vi "SerialPort_MicroZed.vi"(2 "error in (no error)":errorcluster, 3 "COM Port":refnum<visa-resource-name>="COM4") -> (0 "error out":errorcluster)   [LabVIEW 2014]
uses:
  <vilib>/Instr/_visa.llb/VISA Open Access Mode.ctl
  <vilib>/Instr/_visa.llb/VISA Configure Serial Port (Instr).vi
  g_Stop.vi
  g_MicroZed_Interface.vi
  g_ReportControl.vi
panel:
  out "sent":string
  out "Terminal":string
  out "Write":string
  out "read buffer":string
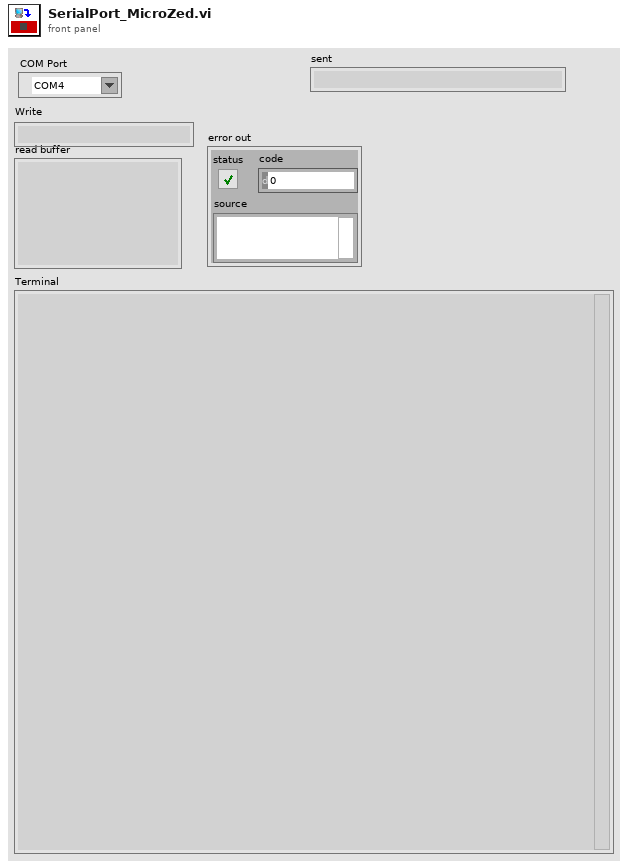
[diagram p1: front panel]
types:
  T1 = typedef "VISA Open Access Mode.ctl" = u32
  T2 = typedef "c_MicroZedInstr_Enum.ctl" = enum16{"Start Test Procedure", "Print Instructions", "Config HCC Register", "Send Parameters"}
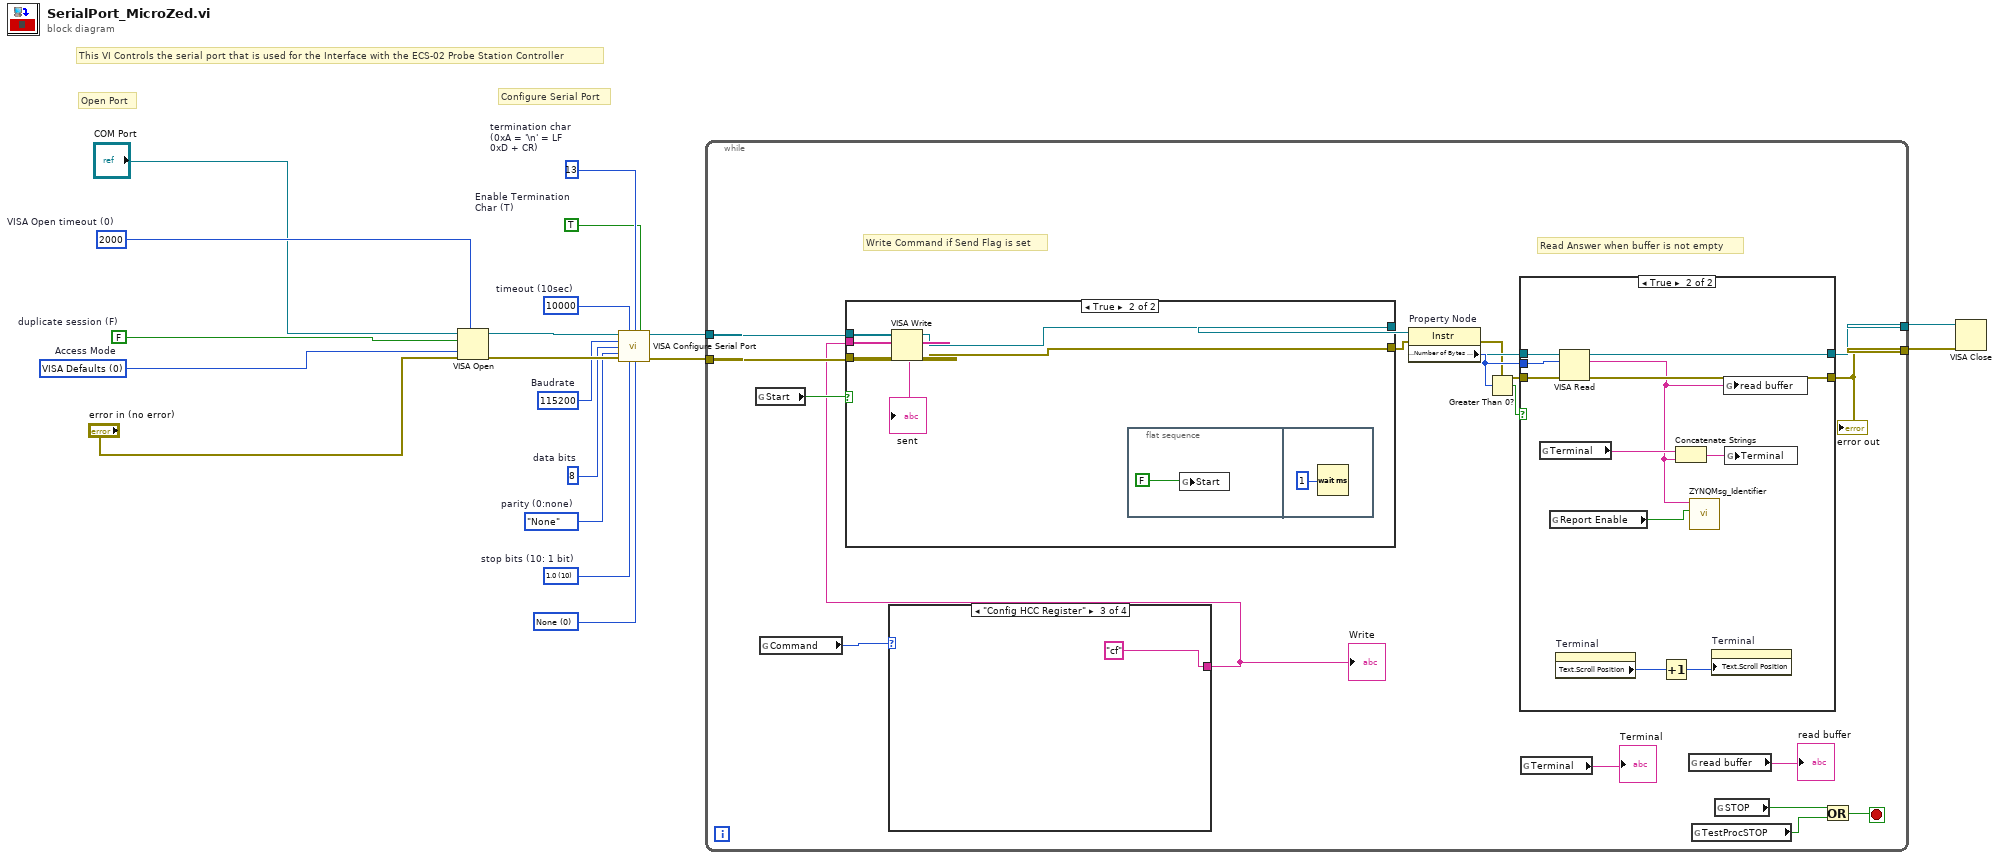
[diagram p0: block diagram]
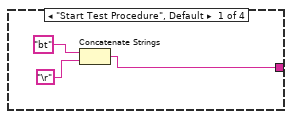
[diagram p2: hidden frame]
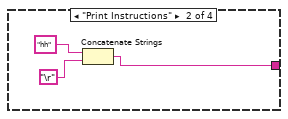
[diagram p3: hidden frame]
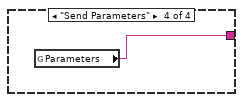
[diagram p4: hidden frame]
diagram:
  w5 = u32 10000  # timeout (10sec)
  w6 = T1 0 items=["VISA Defaults"=0, "Exclusive Lock"=1, "Load Configured Settings"=4]  # Access Mode
  w7 = FALSE  # duplicate session (F)
  w10 = TRUE  # Enable Termination Char (T)
  w11 = u8 13  # termination char (0xA = '\n' = LF 0xD + CR)
  w12 = u16 0 items=["None", "XON/XOFF", "RTS/CTS", "XON/XOFF & RTS/CTS", "DTR/DSR", "XON/XOFF & DTR/DSR"] ("flow control (0:none)")
  w13 = u16 10 items=["1.0"=10, "1.5"=15, "2.0"=20]  # stop bits (10: 1 bit)
  w14 = enum16{"None", "Odd", "Even", "Mark", "Space"}."None"  # parity (0:none)
  w15 = u32 115200  # Baudrate
  w16 = u16 8  # data bits
  w18 = u32 2000  # VISA Open timeout (0)
  # "Configure Serial Port"
  # "This VI Controls the serial port that is used for the Interface with the ECS-02 Probe Station Controller"
  # "Open Port"
  n1 = VISA Open(timeout (0)=w18, duplicate session (F)=w7, access mode=w6, error in (no error)="error in (no error)", VISA resource name="COM Port") -> (VISA resource name=w19:refnum<visa-resource-name>, error out=w17:errorcluster)
  n2 = call-poly "VISA Configure Serial Port"("VISA resource name"=w19, "timeout (10sec)"=w5, "termination char\n(0xA = '\\n' = LF)"=w11, "Enable Termination\nChar (T)"=w10, "baud rate (9600)"=w15, "data bits (8)"=w16, "parity (0:none)"=w14, "error in (no error)"=w17, "stop bits (10: 1 bit)"=w13, "flow control (0:none)"=w12) -> ("VISA resource name out"=w9:refnum<visa-resource-name>, "error out"=w8:errorcluster)  [unwired: 4 in]
  n3 = while {
    tunnel: w9 -> [w35]
    tunnel: w8 -> [w34]
    tunnel: [w36] -> w4
    tunnel: [w37] -> w3
    stop <- w22 stop-if-true
    # "Read Answer when buffer is not empty"
    # "Write Command if Send Flag is set"
    n4 = global read "g_MicroZed_Interface.vi" "Start"() -> (w27:bool)
    n5 = global read "g_MicroZed_Interface.vi" "Command"() -> (w26:T2)
    n6 = case shown="\"Config HCC Register\"" w26 {
      tunnel: [w40 w41 "cf" ("string") w45] -> w25
      frame "Start Test Procedure", Default {
        n7 = Concatenate Strings("bt" ("string"), "\r") -> (w40:string)
      }
      frame "Print Instructions" {
        n8 = Concatenate Strings("hh" ("string"), "\r") -> (w41:string)
      }
      frame "Config HCC Register" {
      }
      frame "Send Parameters" {
        n9 = global read "g_MicroZed_Interface.vi" "Parameters"() -> (w45:string)
      }
    }
    "Write" <- w25
    n10 = case shown="True" w27 {
      tunnel: w35 -> [w59 w65]
      tunnel: w34 -> [w60 w63]
      tunnel: w25 -> [_ w64]
      tunnel: [w60 w61] -> w29
      tunnel: [w59 w62] -> w30
      frame False {
      }
      frame True {
        n11 = VISA Write(VISA resource name=w65, write buffer=w64, error in (no error)=w63) -> (VISA resource name out=w62:refnum<visa-resource-name>, error out=w61:errorcluster)  [unwired: 1 out]
        n12 = flat-sequence {
          frame #0 {
            n13 = global write "g_MicroZed_Interface.vi" "Start"(FALSE ("Start")) -> ()
          }
          frame #1 {
            n14 = Wait (ms)(milliseconds to wait=u32 1) -> ()  [unwired: 1 out]
          }
        }
        "sent" <- w64
      }
    }
    n15 = property on="Property Node" class="Instr"(reference=w30, error in=w29) -> (reference out=w31:refnum<visa-resource-name>, error out=w28:errorcluster, "Serial Settings:Number of Bytes at Serial Port"=w32:u32)
    n16 = Greater Than 0?(x=w32) -> (x > 0?=w33:bool)
    n17 = case shown="True" w33 {
      tunnel: w31 -> [w47 w58]
      tunnel: w28 -> [w46 w57]
      tunnel: [w47 w56] -> w37
      tunnel: [w46 w55] -> w36
      tunnel: w32 -> [_ w54]
      frame False {
      }
      frame True {
        n18 = global read "g_MicroZed_Interface.vi" "Terminal"() -> (w51:string)
        n19 = global read "g_ReportControl.vi" "Report Enable"() -> (w48:bool)
        n20 = property on="Terminal" class="Str"() -> ("Text.Scroll Position"=w53:u32)  [unwired: 2 in, 2 out]
        n21 = VISA Read(VISA resource name=w58, byte count=w54, error in (no error)=w57) -> (VISA resource name out=w56:refnum<visa-resource-name>, read buffer=w49:string, error out=w55:errorcluster)  [unwired: 1 out]
        n22 = Increment(x=w53) -> (x+1=w52:u32)
        n23 = Concatenate Strings(w51, w49) -> (w50:string)
        n24 = call "ZYNQMsg_Identifier.vi"("Enable"=w48, "Message"=w49) -> ()  [unwired: 10 in]
        n25 = property on="Terminal" class="Str"("Text.Scroll Position"=w52) -> ()  [unwired: 2 in, 2 out]
        n26 = global write "g_MicroZed_Interface.vi" "read buffer"(w49) -> ()
        n27 = global write "g_MicroZed_Interface.vi" "Terminal"(w50) -> ()
      }
    }
    "error out" <- w36
    n28 = global read "g_MicroZed_Interface.vi" "Terminal"() -> (→"Terminal":string)
    n29 = global read "g_MicroZed_Interface.vi" "read buffer"() -> (→"read buffer":string)
    n30 = global read "g_Stop.vi" "TestProcSTOP"() -> (w20:bool)
    n31 = global read "g_Stop.vi" "STOP"() -> (w21:bool)
    n32 = Or(x=w21, y=w20) -> (x .or. y?=w22:bool)
  }
  n33 = VISA Close(VISA resource name=w3, error in (no error)=w4) -> ()  [unwired: 1 out]
